vi "Interface 1.vi"() -> ()   [LabVIEW 2013]
panel:
  in  "stop":bool
  in  "Enter the sensor node URL":string[](array[string])=["C:\\Users\\OverCrash\\Dropbox\\projeto_DragonBoard410C\\Labview\\SensorNode_index.html"]
  out "Sensor data":T1(array[cluster])=[{"Temperature [ºC] "=23.0, "Distance [cm]"=184.0, "Battery [mV]"=2746.0, "Sensor ID"=">SENSORNODE 01<", "Uptime"=33.0}] {"Uptime" format="%<%H:%M:%S>t"; "Distance [cm]" scale=0.0..200.0; "Temperature [ºC]" scale=0.0..100.0}
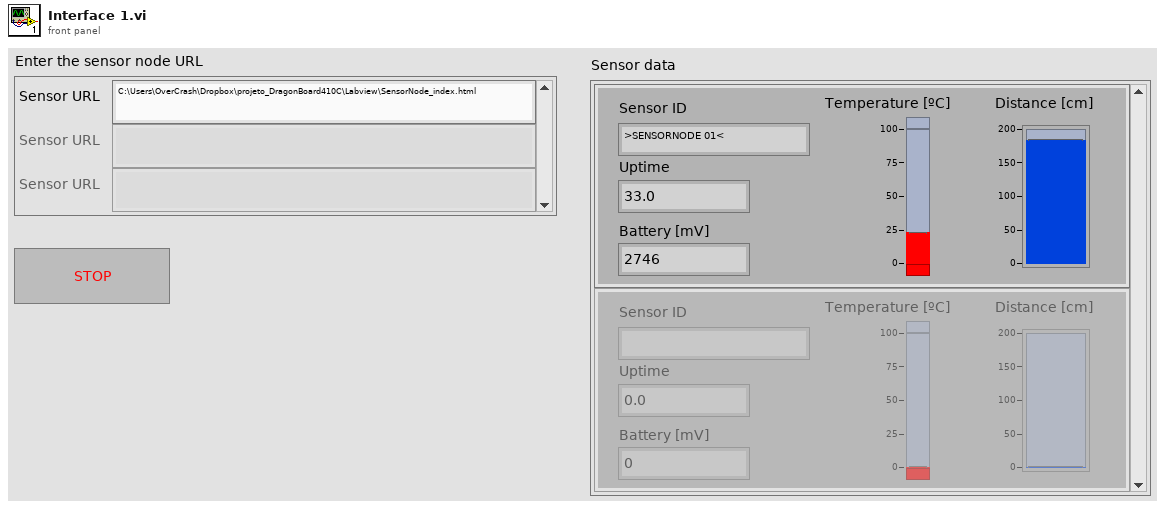
[diagram p1: front panel]
types:
  T1 = cluster{"Temperature [ºC] ":dbl, "Distance [cm]":dbl, "Battery [mV]":dbl, "Sensor ID":string, "Uptime":dbl}[]
  T2 = cluster{"Temperature [ºC] ":dbl, "Distance [cm]":dbl, "Battery [mV]":dbl, "Sensor ID":string, "Uptime":dbl}
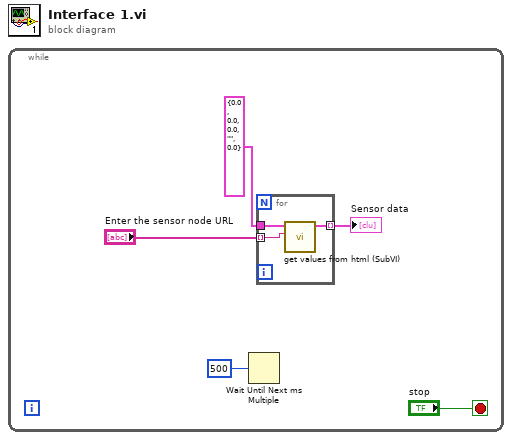
[diagram p0: block diagram]
diagram:
  n1 = while {
    stop <- "stop" stop-if-true
    n2 = Wait Until Next ms Multiple(millisecond multiple=u32 500) -> ()  [unwired: 1 out]
    n3 = for {
      tunnel: "Enter the sensor node URL" -> [w8] mode=indexing
      tunnel: T2 {"Temperature [ºC] "=0.0, "Distance [cm]"=0.0, "Battery [mV]"=0.0, "Sensor ID"="", "Uptime"=0.0} ("Cluster") -> [w7]
      tunnel: [w6] -> w3 mode=indexing
      n4 = call "get values from html (SubVI).vi"("Sensor URL"=w8, "Cluster in"=w7) -> ("Cluster out"=w6:T2)  [unwired: 9 in]
    }
    "Sensor data" <- w3
  }
